vi "ICNC Move Profile Rel Async.vi"(5 "Distance":i32, 6 "Decel":u32, 7 "Speed":u32, 8 "error in (no error)":errorcluster caption="entrée d'erreur (pas d'erreur)", 9 "Accel":u32, 10 "FStartStop":u32, 11 "Axe":u32) -> (0 "error out":errorcluster caption="sortie d'erreur", 3 "function return":u32)   [LabVIEW 2012, in "ICNC2.lvlib"]
doc: "DWORD ICNC_MoveProfileRelAsync( DWORD Axe,\n DWORD FStartStop,\n DWORD Accel,\n DWORD Speed,\n DWORD Decel,\n INT Distance);"
uses:
  <userlib>/ICNC/ICNC2.lvlib
  <userlib>/ICNC/ICNC2.dll
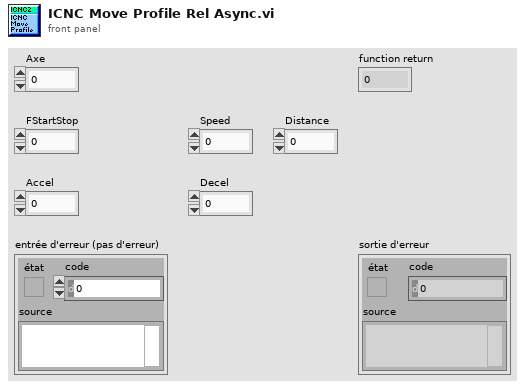
[diagram p1: front panel]
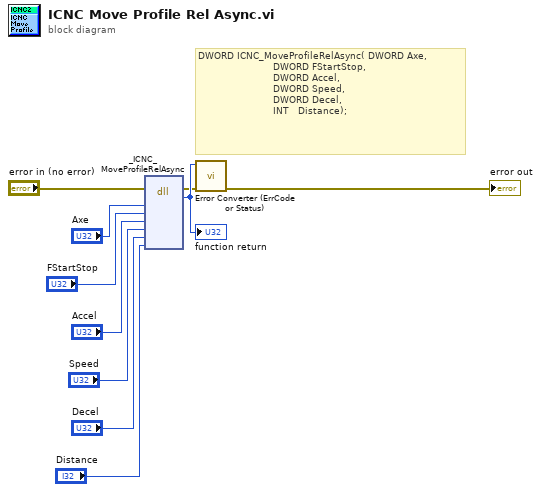
[diagram p0: block diagram]
diagram:
  # "DWORD ICNC_MoveProfileRelAsync( DWORD Axe,\n                         DWORD FStartStop,\n                         DWORD Accel,\n                         DWORD Speed,\n                         DWORD Decel,\n                         INT   Distance);"
  n1 = dll-call lib="C:/Program Files (x86)/National Instruments/LabVIEW 2012/user.lib/ICNC/ICNC2.*" fn="_ICNC_MoveProfileRelAsync"(error in="error in (no error)", "Axe"="Axe", "FStartStop"="FStartStop", "Accel"="Accel", "Speed"="Speed", "Decel"="Decel", "Distance"="Distance") -> (error out=w2:errorcluster, w10:u32)  [unwired: 8 in, 1 out]
  "function return" <- w10
  n2 = call <userlib>:"Error Converter (ErrCode or Status).vi"("error in (no error)"=w2, "error code"=w10) -> ("error out"=→"error out":errorcluster)  [unwired: 9 in]
